vi "Ini key write (Boolean).vi"(7 "Section":string, 8 "error in (no error)":errorcluster, 9 "Values (Boolean)":bool[](array[boolean]), 10 "Ini file interface":T2, 11 "Ini file refnum in":T1) -> (0 "error out":errorcluster, 3 "Ini file refnum out":T1)   [LabVIEW 2013]
uses:
  <vilib>/Utility/config.llb/Config Data RefNum.ctl
  Typedefs/Ini file interface (Boolean).ctl
  <vilib>/Utility/config.llb/Read Key (Boolean).vi
  <vilib>/Utility/config.llb/Write Key (Boolean).vi
  <vilib>/Utility/config.llb/NI_LVConfig.lvlib
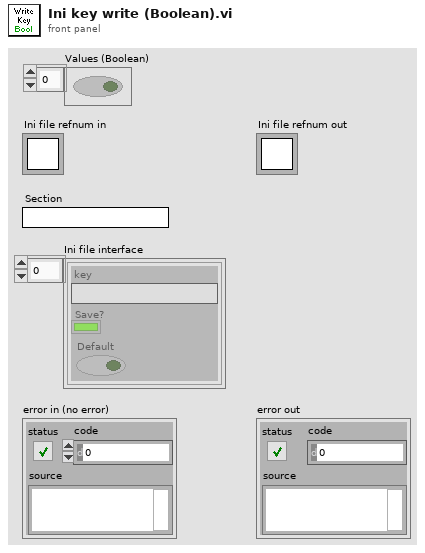
[diagram p1: front panel]
types:
  T1 = typedef "NI_LVConfig.lvlib/Config Data RefNum.ctl" = refnum<k1>
  T2 = typedef "Ini file interface (Boolean).ctl" = cluster{"key":string, "Save?":bool, "Default":bool}[]
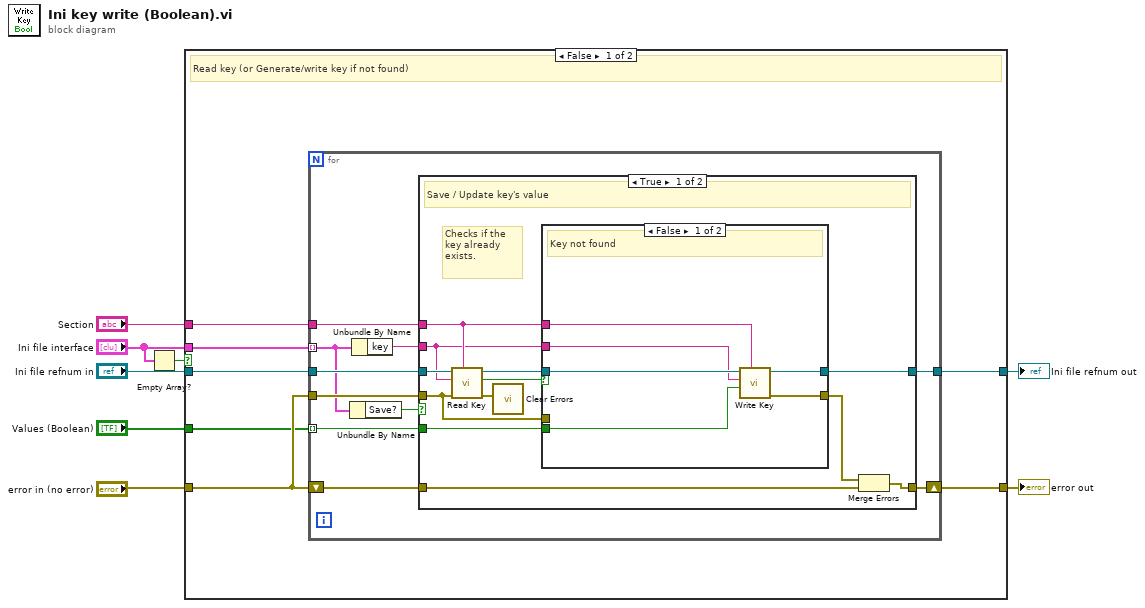
[diagram p0: block diagram]
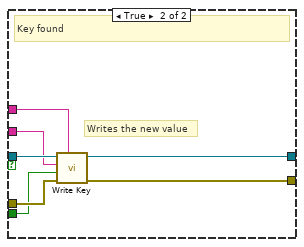
[diagram p2: hidden frame]
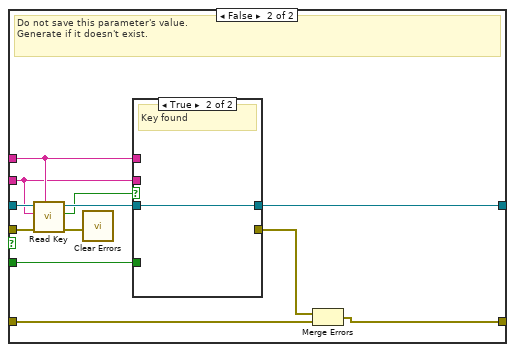
[diagram p3: hidden frame]
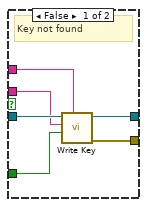
[diagram p4: hidden frame]
diagram:
  n1 = Empty Array?(array="Ini file interface") -> (empty?=w3:bool)
  n2 = case shown="False" w3 {
    tunnel: "Ini file refnum in" -> [w15 w71]
    tunnel: [w14 w71] -> w8
    tunnel: [w13 w70] -> w7
    tunnel: "error in (no error)" -> [w12 w70]
    tunnel: "Section" -> [w9 _]
    tunnel: "Ini file interface" -> [w11 _]
    tunnel: "Values (Boolean)" -> [w10 _]
    frame False {
      # "Read key (or Generate/write key if not found)"
      n3 = for {
        tunnel: w15 -> [w25]
        tunnel: w12 -> [w24]
        tunnel: [w23] -> w14
        shift-right: [w22] -> w13
        shift-left: w12 -> [w21]
        tunnel: w11 -> [w17] mode=indexing
        tunnel: w10 -> [w20] mode=indexing
        tunnel: w9 -> [w19]
        n4 = Unbundle By Name(w17) -> ("Save?"=w16:bool)
        n5 = Unbundle By Name(w17) -> ("key"=w18:string)
        n6 = case shown="True" w16 {
          tunnel: w25 -> [w37 w62]
          tunnel: w24 -> [w26 w61]
          tunnel: [w28 w52] -> w23
          tunnel: [w36 w60] -> w22
          tunnel: w21 -> [w35 w59]
          tunnel: w18 -> [w31 w55]
          tunnel: w20 -> [w29 w53]
          tunnel: w19 -> [w32 w56]
          frame True {
            # "Checks if the key already exists."
            # "Save / Update key's value"
            n7 = call-poly <vilib>:"Read Key.vi"("section"=w32, "error in (no error)"=w26, "key"=w31, "refnum"=w37) -> ("error out"=w34:errorcluster, "found?"=w27:bool, "refnum out"=w33:T1)  [unwired: 4 in, 1 out]
            n8 = call <vilib>:"Clear Errors.vi"("error in (no error)"=w34) -> ()  [unwired: 6 in, 1 out]
            n9 = case shown="False" w27 {
              tunnel: w33 -> [w43 w50]
              tunnel: [w42 w49] -> w28
              tunnel: [w41 w47] -> w30
              tunnel: w32 -> [w40 w46]
              tunnel: w31 -> [w38 w45]
              tunnel: w29 -> [w39 w44]
              tunnel: w26 -> [_ w48]
              frame False {
                # "Key not found"
                n10 = call-poly <vilib>:"Write Key.vi"("section"=w40, "value"=w39, "key"=w38, "refnum"=w43) -> ("error out"=w41:errorcluster, "refnum out"=w42:T1)  [unwired: 5 in, 1 out]
              }
              frame True {
                # "Writes the new value"
                # "Key found"
                n11 = call-poly <vilib>:"Write Key.vi"("section"=w46, "error in (no error)"=w48, "value"=w44, "key"=w45, "refnum"=w50) -> ("error out"=w47:errorcluster, "refnum out"=w49:T1)  [unwired: 4 in, 1 out]
              }
            }
            n12 = Merge Errors(w30, w35) -> (w36:errorcluster)
          }
          frame False {
            # "Do not save this parameter's value.\nGenerate if it doesn't exist."
            n13 = call-poly <vilib>:"Read Key.vi"("section"=w56, "error in (no error)"=w61, "key"=w55, "refnum"=w62) -> ("error out"=w58:errorcluster, "found?"=w51:bool, "refnum out"=w57:T1)  [unwired: 4 in, 1 out]
            n14 = call <vilib>:"Clear Errors.vi"("error in (no error)"=w58) -> ()  [unwired: 6 in, 1 out]
            n15 = case shown="True" w51 {
              tunnel: w57 -> [w68 w69]
              tunnel: [w67 w69] -> w52
              tunnel: [w66 _] -> w54
              tunnel: w56 -> [w65 _]
              tunnel: w55 -> [w64 _]
              tunnel: w53 -> [w63 _]
              frame False {
                # "Key not found"
                n16 = call-poly <vilib>:"Write Key.vi"("section"=w65, "value"=w63, "key"=w64, "refnum"=w68) -> ("error out"=w66:errorcluster, "refnum out"=w67:T1)  [unwired: 5 in, 1 out]
              }
              frame True {
                # "Key found"
              }
            }
            n17 = Merge Errors(w54, w59) -> (w60:errorcluster)
          }
        }
      }
    }
    frame True {
      # "Setup array is empty"
    }
  }
  "Ini file refnum out" <- w8
  "error out" <- w7
